vi "Lookup Descendants.vi"(8 "error in (no error)":errorcluster, 10 "Lookup":refnum<class "Config Lookup.lvclass">, 11 "VolatusConfigElement in":refnum<class "VolatusConfigElement.lvclass">) -> (0 "error out":errorcluster, 2 "Descendants":refnum<class "Config Element.lvclass">[](array[class]), 3 "VolatusConfigElement out":refnum<class "VolatusConfigElement.lvclass">)   [LabVIEW 2020, in "VolatusConfig.lvlib" / "VolatusConfigElement.lvclass"]
uses:
  VolatusConfigElement.lvclass
  lv-cdm/CDM-Config/Config Filter/Config Lookup.lvclass
  lv-cdm/CDM-Config/Config Element/Config Element.lvclass
  VolatusConfigElement.lvclass/VolatusConfigElement.ctl
  lv-cdm/CDM-Config/Config Element/Owner.vi
  lv-cdm/CDM-Config/Config Manager/Lookup Descendant.vi
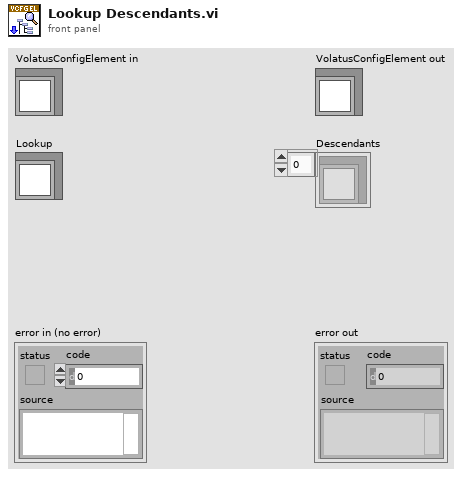
[diagram p1: front panel]
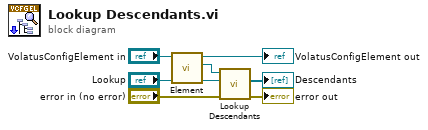
[diagram p0: block diagram]
diagram:
  n1 = call "Element.vi"("VolatusConfigElement in"="VolatusConfigElement in") -> ("Element"=w5:refnum<class "Config Element.lvclass">, "VolatusConfigElement out"=→"VolatusConfigElement out":refnum<class "VolatusConfigElement.lvclass">)  [unwired: 9 in]
  n2 = call "Lookup Descendants.vi"("error in (no error)"="error in (no error)", "Lookup"="Lookup", "Config Element in"=w5) -> ("error out"=→"error out":errorcluster, "Descendants"=→"Descendants":refnum<class "Config Element.lvclass">[])  [unwired: 6 in, 1 out]
